vi "FGV Gasbottledefinition.vi"(6 "Aktion":T5, 8 "error in (no error)":errorcluster caption="Fehler (Eingang, kein Fehler)", 11 "Gasflasche Text Array":T3[](array[typedef])) -> (0 "error out":errorcluster caption="Fehler (Ausgang)", 2 "Gasflaschen Liste gesamt":T1[](array[typedef]) {"Gasflasche"."Ablaufdatum" format="%<%d.%m.%Y>T"; "Komponenten"."Konzentration IST" format="%#.4f"; "Komponenten"."Genauigkeit" format="%#.1f"}, 3 "Gasflaschen Text Liste gesamt":T3[][](array[typedef]))   [LabVIEW 2020, in "System Einstellungen V2.lvlib"]
uses:
  System Einstellungen V2.lvlib
  Aktion FGV Gasbottledefinition.ctl
  Traegergas.ctl
  Gasflasche gesamt.ctl
  Gasflasche.ctl
  Gasflaschenkomponente.ctl
  EPA 1065/Allgemeine VIs/Aktion Wertaenderung Gasliste.ctl
  Allgemein/allgemeine Sub-VIs.lvlib
  EPA 1065/EPA 1065.lvlib
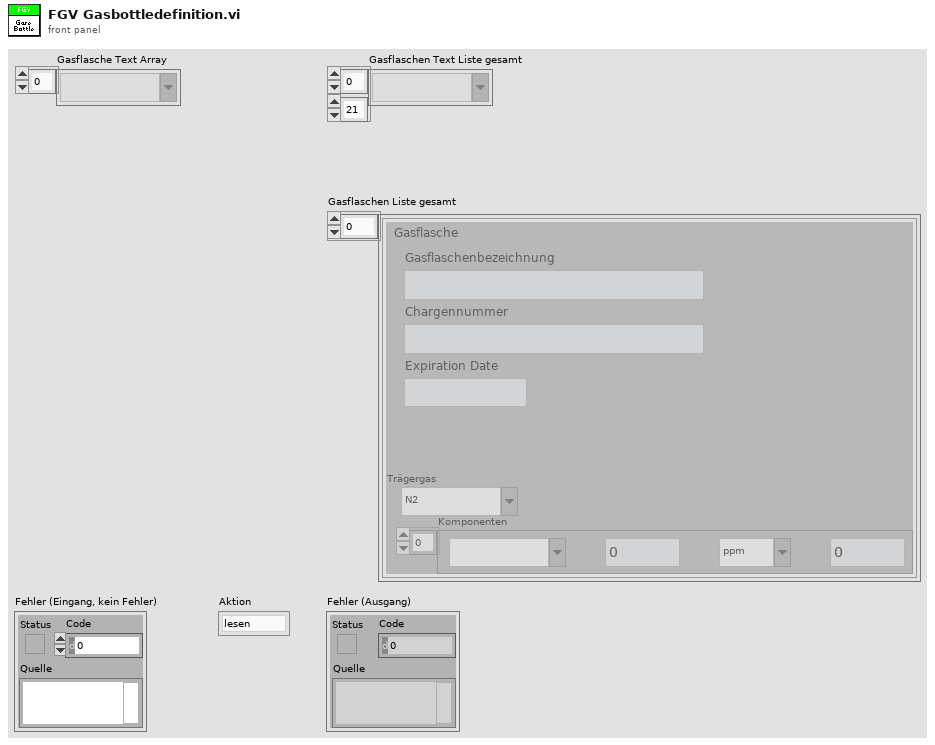
[diagram p1: front panel]
types:
  T1 = typedef "System Einstellungen V2.lvlib/Gasflasche gesamt.ctl" = cluster{"Gasflasche":T2, "Trägergas":T3, "Komponenten":T4[]}
  T2 = typedef "System Einstellungen V2.lvlib/Gasflasche.ctl" = cluster{"Gasname für die Auswahl":string, "Chargennummer":string, "Ablaufdatum":timestamp}
  T3 = typedef "System Einstellungen V2.lvlib/Traegergas.ctl" = string
  T4 = typedef "System Einstellungen V2.lvlib/Gasflaschenkomponente.ctl" = cluster{"Gasauswahl":string, "Konzentration IST":dbl, "Einheit":string, "Genauigkeit":dbl}
  T5 = typedef "System Einstellungen V2.lvlib/Aktion FGV Gasbottledefinition.ctl" = enum16{"lesen", "schreiben", "löschen", "laden", "speichern", "exportieren", "importieren"}
  T6 = typedef "EPA 1065.lvlib/Aktion Wertaenderung Gasliste.ctl" = enum16{"Init", "lesen", "Gasliste geändert", "ARN inaktiv", "LEAK inaktiv", "Interference 366 inaktiv", "T90 inaktiv", "Interference 375 inaktiv", "Chiller inaktiv", "FID O2 inaktiv", "FID Opti inaktiv", "Drift inaktiv", "Pre Test inaktiv", "LinV2 inaktiv"}
  T7 = enum16{"lesen", "schreiben", "löschen", "laden", "speichern"}
  T8 = enum16{"open", "replace", "create", "open or create", "replace or create", "replace or create with confirmation"}
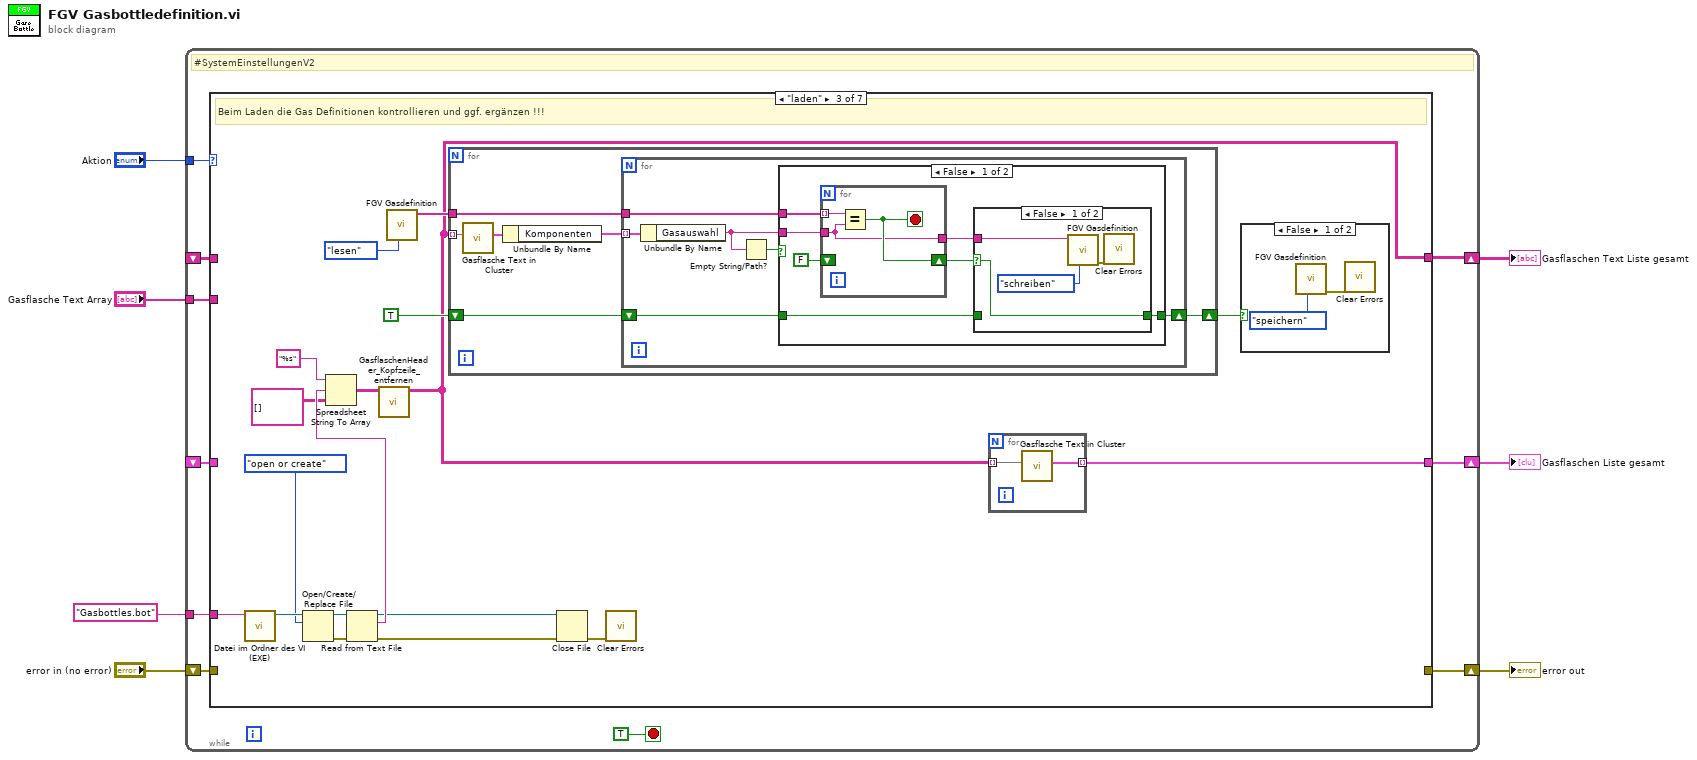
[diagram p0: block diagram]
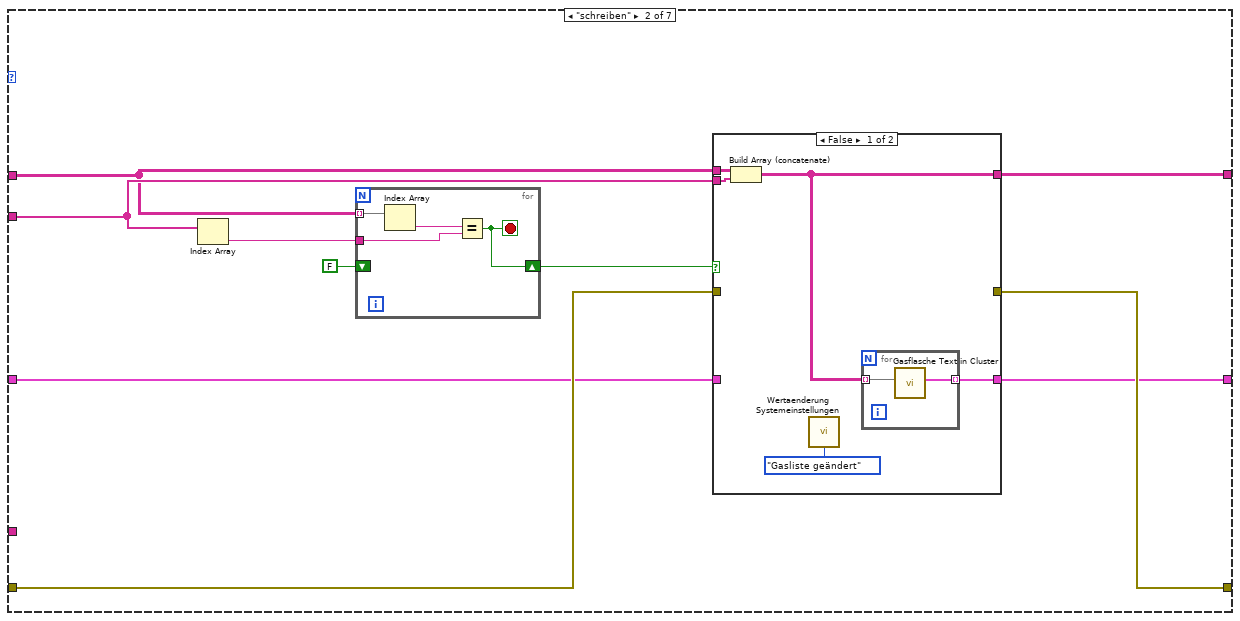
[diagram p3: hidden frame]
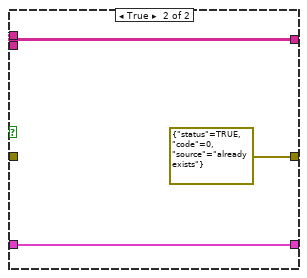
[diagram p4: hidden frame]
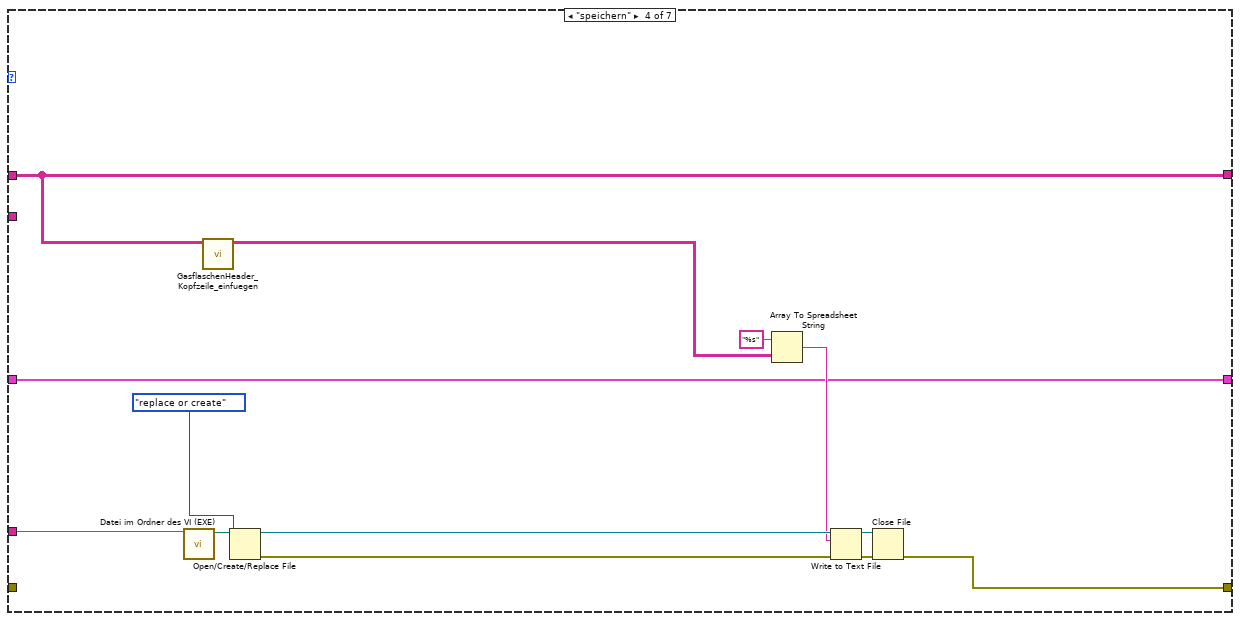
[diagram p8: hidden frame]
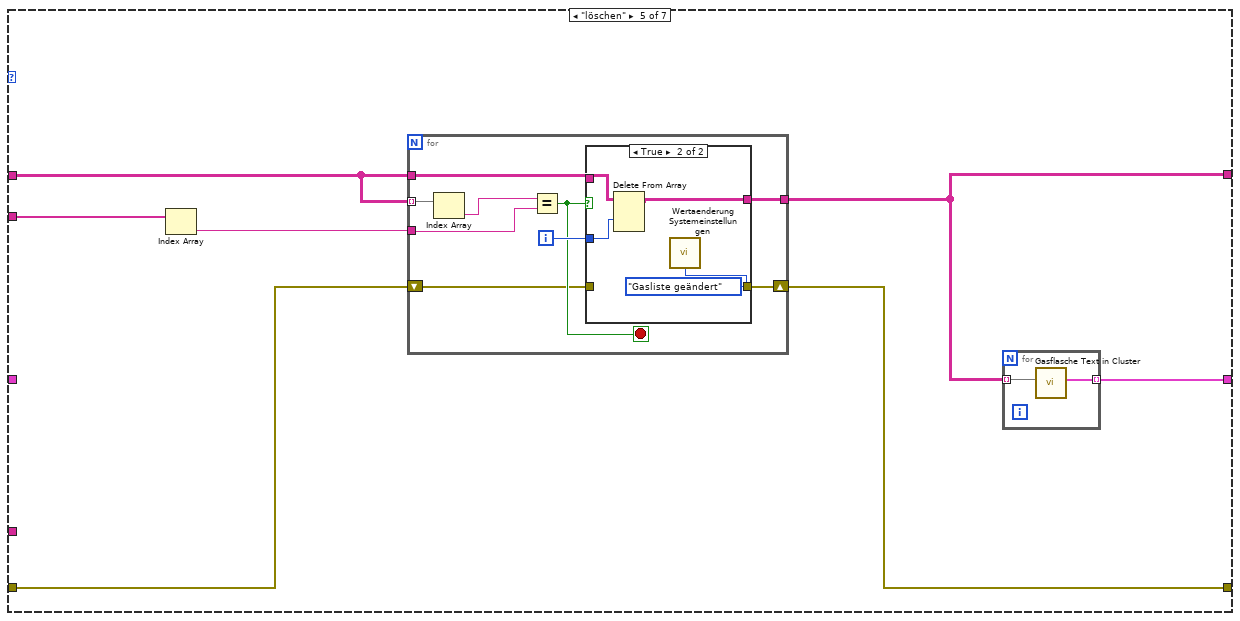
[diagram p9: hidden frame]
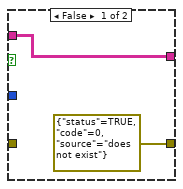
[diagram p10: hidden frame]
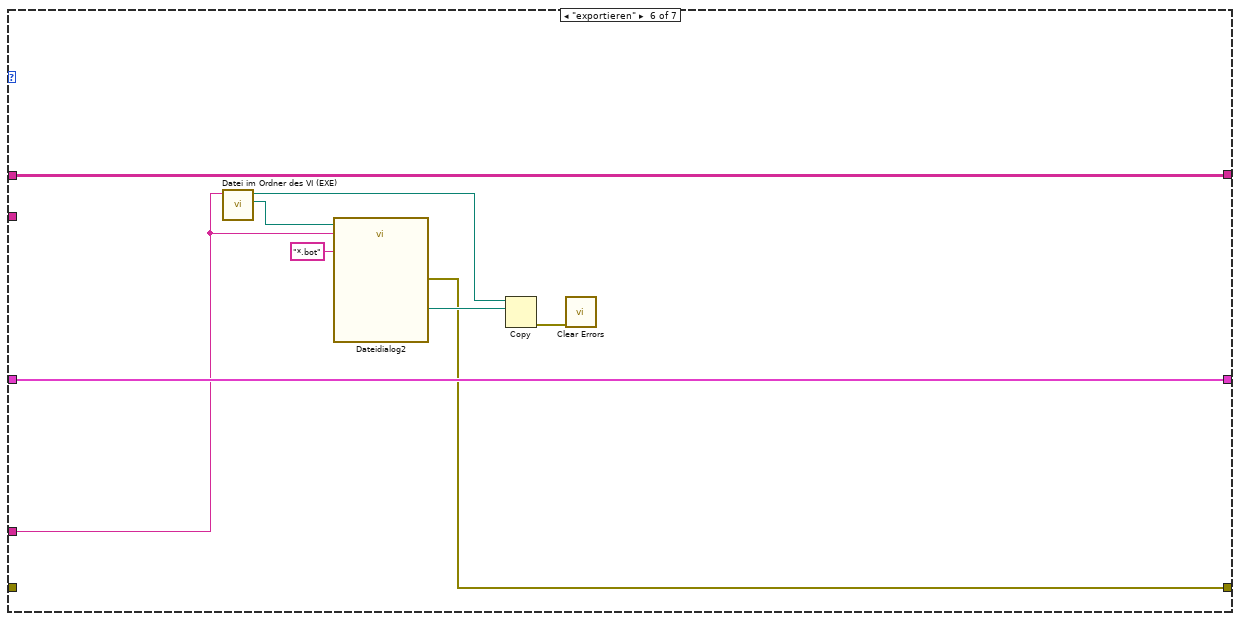
[diagram p11: hidden frame]
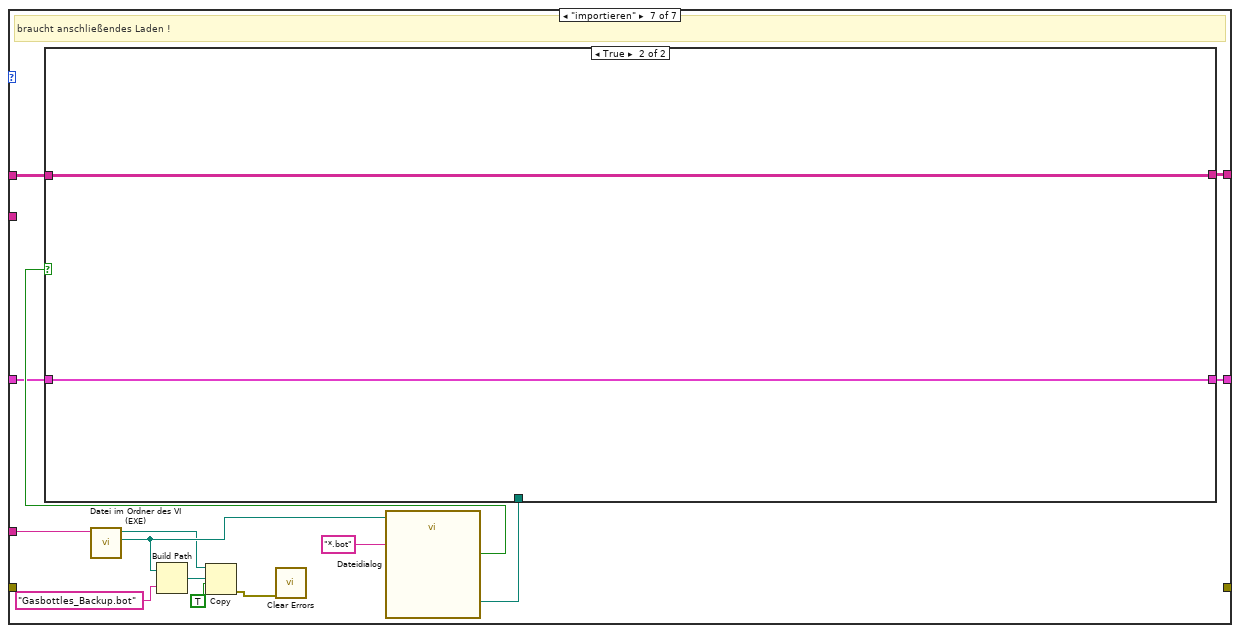
[diagram p12: hidden frame]
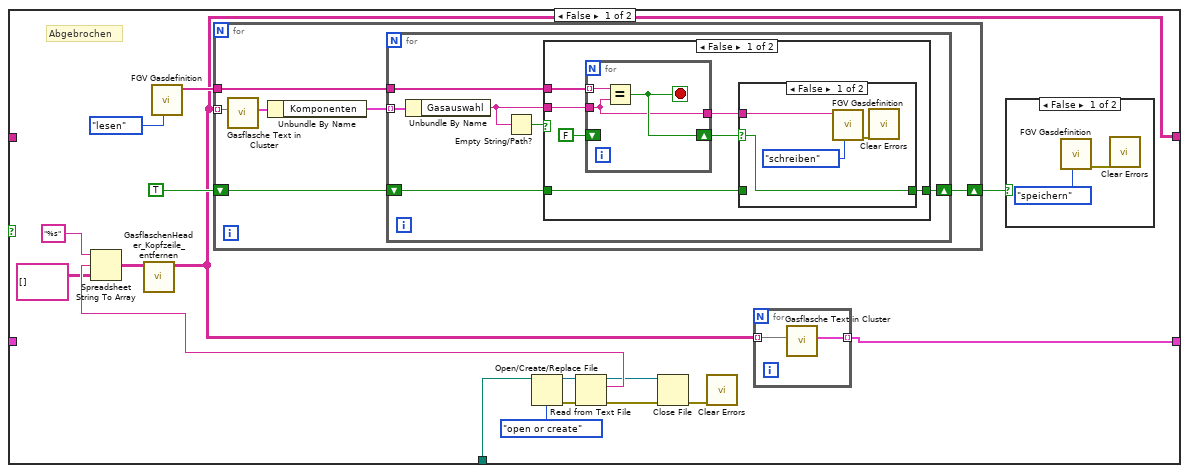
[diagram p13: hidden frame]
diagram:
  n1 = while {
    tunnel: "Aktion" -> [w16]
    shift-right: [w13] -> w2
    shift-left: _ -> [w15]
    tunnel: "Gasbottles.bot" ("Dateiname") -> [w14]
    tunnel: "Gasflasche Text Array" -> [w12]
    shift-right: [w10] -> w3
    shift-left: "error in (no error)" -> [w11]
    shift-right: [w9] -> w1
    shift-left: _ -> [w8]
    stop <- TRUE stop-if-true
    # "#SystemEinstellungenV2"
    n2 = case shown="\"laden\"" w16 {
      tunnel: [w19 w29 w45 w95 w108 w139 w151] -> w13
      tunnel: w15 -> [w19 w24 _ w95 w111 w139 w141]
      tunnel: w14 -> [_ _ w61 w105 _ w132 w153]
      tunnel: w12 -> [_ w26 _ _ w113 _ _]
      tunnel: w11 -> [_ w23 _ _ w110 _ _]
      tunnel: [_ w22 _ w97 w109 w133 _] -> w10
      tunnel: [w18 w21 w46 w96 w107 w138 w150] -> w9
      tunnel: w8 -> [w18 w20 _ w96 _ w138 w140]
      frame "lesen", Default {
      }
      frame "schreiben" {
        n3 = Index Array(array=w26) -> (element=w25:T3)  [unwired: 1 in]
        n4 = for {
          tunnel: w25 -> [w43]
          shift-right: [w42] -> w27
          shift-left: FALSE -> [_]
          tunnel: w24 -> [w41] mode=indexing
          stop <- w42 stop-if-true
          n5 = Index Array(array=w41) -> (element=w40:T3)  [unwired: 1 in]
          n6 = Equal?(x=w40, y=w43) -> (x = y?=w42:bool)
        }
        n7 = case shown="False" w27 {
          tunnel: [w32 w39] -> w29
          tunnel: w24 -> [w34 w39]
          tunnel: w26 -> [w33 _]
          tunnel: w23 -> [_ _]
          tunnel: [_ errorcluster {"status"=TRUE, "code"=0, "source"="already exists"} ("error in (no error)")] -> w22
          tunnel: [w31 w37] -> w21
          tunnel: w20 -> [_ w37]
          frame False {
            n8 = Build Array (concatenate)(w34, w33) -> (w32:T3[][])
            n9 = call "Wertaenderung Systemeinstellungen.vi"("Aktion"=Aktion_Wertaenderung_Gasliste."Gasliste geändert") -> ()  [unwired: 13 in, 2 out]
            n10 = for {
              tunnel: w32 -> [w36] mode=indexing
              tunnel: [w35] -> w31 mode=indexing
              n11 = call "Gasflasche Text in Cluster.vi"("Gasflasche Text Array"=w36) -> ("Gasflasche"=w35:T1)  [unwired: 10 in]
            }
          }
          frame True {
          }
        }
      }
      frame "laden" {
        # "Beim Laden die Gas Definitionen kontrollieren und ggf. ergänzen !!!"
        n12 = call "Datei im Ordner des VI (EXE).vi"("Dateiname"=w61) -> ("Dateipfad im Ordner des Haupt-VIs"=w60:path)  [unwired: 8 in, 2 out]
        n13 = Open/Create/Replace File(file path (use dialog)=w60, operation (0:open)=T8."open or create" ("Operation (0:open)")) -> (refnum out=w58:refnum<file>, error out=w59:errorcluster)  [unwired: 4 in, 1 out]
        n14 = Read from Text File(file (use dialog)=w58, error in=w59) -> (refnum out=w54:refnum<file>, text=w57:string, error out=w53:errorcluster)  [unwired: 2 in, 1 out]
        n15 = Spreadsheet String To Array(format string="%s" ("Format-String"), spreadsheet string=w57, array type (2D Dbl)=string[][] []) -> (array=w44:string[][])  [unwired: 1 in]
        n16 = call "GasflaschenHeader_Kopfzeile_entfernen.vi"("Array (Eingang)"=w44) -> ("Array (Ausgang)"=w45:string[][])  [unwired: 10 in]
        n17 = call "FGV Gasdefinition.vi"("Aktion"=T7."lesen") -> ("Gase"=w49:string[])  [unwired: 9 in, 1 out]
        n18 = for {
          tunnel: w45 -> [w68] mode=indexing
          tunnel: w49 -> [w71]
          shift-right: [w69] -> w47
          shift-left: TRUE -> [w70]
          n19 = call "Gasflasche Text in Cluster.vi"("Gasflasche Text Array"=w68) -> ("Gasflasche"=w67:T1)  [unwired: 10 in]
          n20 = Unbundle By Name(w67) -> ("Komponenten"=w66:T4[])
          n21 = for {
            tunnel: w71 -> [w77]
            tunnel: w66 -> [w74] mode=indexing
            shift-right: [w75] -> w69
            shift-left: w70 -> [w76]
            n22 = Unbundle By Name(w74) -> ("Gasauswahl"=w72:string)
            n23 = Empty String/Path?(string/path=w72) -> (empty?=w73:bool)
            n24 = case shown="False" w73 {
              tunnel: w77 -> [w84 _]
              tunnel: w76 -> [w80 w93]
              tunnel: [w79 w93] -> w75
              tunnel: w72 -> [w78 _]
              frame False {
                n25 = for {
                  tunnel: w84 -> [w92] mode=indexing
                  tunnel: w78 -> [w90]
                  shift-right: [w91] -> w81
                  shift-left: FALSE -> [_]
                  tunnel: [w90] -> w82
                  stop <- w91 stop-if-true
                  n26 = Equal?(x=w92, y=w90) -> (x = y?=w91:bool)
                }
                n27 = case shown="False" w81 {
                  selector: w81 -> [w86 _]
                  tunnel: w82 -> [w87 _]
                  tunnel: w80 -> [_ w89]
                  tunnel: [w86 w89] -> w79
                  frame False {
                    n28 = call "FGV Gasdefinition.vi"("Aktion"=T7."schreiben", "Gas"=w87) -> ("error out"=w85:errorcluster)  [unwired: 8 in, 1 out]
                    n29 = call <vilib>:"Clear Errors.vi"("error in (no error)"=w85) -> ()  [unwired: 5 in, 2 out]
                  }
                  frame True {
                  }
                }
              }
              frame True {
              }
            }
          }
        }
        n30 = Close File(refnum=w54, error in=w53) -> (error out=w55:errorcluster)  [unwired: 1 out]
        n31 = call <vilib>:"Clear Errors.vi"("error in (no error)"=w55) -> ()  [unwired: 5 in, 2 out]
        n32 = for {
          tunnel: w45 -> [w63] mode=indexing
          tunnel: [w62] -> w46 mode=indexing
          n33 = call "Gasflasche Text in Cluster.vi"("Gasflasche Text Array"=w63) -> ("Gasflasche"=w62:T1)  [unwired: 10 in]
        }
        n34 = case shown="False" w47 {
          frame False {
            n35 = call "FGV Gasdefinition.vi"("Aktion"=T7."speichern") -> ("error out"=w64:errorcluster)  [unwired: 9 in, 1 out]
            n36 = call <vilib>:"Clear Errors.vi"("error in (no error)"=w64) -> ()  [unwired: 5 in, 2 out]
          }
          frame True {
          }
        }
      }
      frame "speichern" {
        n37 = call "Datei im Ordner des VI (EXE).vi"("Dateiname"=w105) -> ("Dateipfad im Ordner des Haupt-VIs"=w106:path)  [unwired: 8 in, 2 out]
        n38 = call "GasflaschenHeader_Kopfzeile_einfuegen.vi"("Array (Eingang)"=w95) -> ("Array (Ausgang)"=w94:T3[][])  [unwired: 10 in]
        n39 = Open/Create/Replace File(file path (use dialog)=w106, operation (0:open)=T8."replace or create" ("Operation (0:open)")) -> (refnum out=w104:refnum<file>, error out=w103:errorcluster)  [unwired: 4 in, 1 out]
        n40 = Array To Spreadsheet String(array=w94, 3:"%s" ("Format-String")) -> (spreadsheet string=w100:string)  [unwired: 1 in]
        n41 = Write to Text File(file (use dialog)=w104, text=w100, error in=w103) -> (refnum out=w101:refnum<file>, error out=w102:errorcluster)  [unwired: 1 in, 1 out]
        n42 = Close File(refnum=w101, error in=w102) -> (error out=w97:errorcluster)  [unwired: 1 out]
      }
      frame "löschen" {
        n43 = Index Array(array=w113) -> (element=w112:T3)  [unwired: 1 in]
        n44 = for {
          tunnel: w112 -> [w124]
          tunnel: w111 -> [w123]
          tunnel: [w121] -> w108
          tunnel: w111 -> [w119] mode=indexing
          shift-right: [w116] -> w109
          shift-left: w110 -> [w117]
          i -> [w122]
          stop <- w120 stop-if-true
          n45 = Index Array(array=w119) -> (element=w118:T3)  [unwired: 1 in]
          n46 = Equal?(x=w118, y=w124) -> (x = y?=w120:bool)
          n47 = case shown="True" w120 {
            tunnel: w123 -> [w126 w130]
            tunnel: w122 -> [_ w129]
            tunnel: [w126 w128] -> w121
            tunnel: w117 -> [_ _]
            tunnel: [errorcluster {"status"=TRUE, "code"=0, "source"="does not exist"} ("error in (no error)") _] -> w116
            frame False {
            }
            frame True {
              n48 = Delete From Array(array=w130, index (row)=w129) -> (array with subset deleted=w128:T3[][])  [unwired: 2 in, 1 out]
              n49 = call "Wertaenderung Systemeinstellungen.vi"("Aktion"=Aktion_Wertaenderung_Gasliste."Gasliste geändert") -> ()  [unwired: 13 in, 2 out]
            }
          }
        }
        n50 = for {
          tunnel: w108 -> [w115] mode=indexing
          tunnel: [w114] -> w107 mode=indexing
          n51 = call "Gasflasche Text in Cluster.vi"("Gasflasche Text Array"=w115) -> ("Gasflasche"=w114:T1)  [unwired: 10 in]
        }
      }
      frame "exportieren" {
        n52 = call "Datei im Ordner des VI (EXE).vi"("Dateiname"=w132) -> ("Ordner des Haupt-VIs"=w137:path, "Dateipfad im Ordner des Haupt-VIs"=w135:path)  [unwired: 8 in, 1 out]
        n53 = call "Dateidialog2"("start path"=w137, "default name"=w132, "pattern (all files)"="*.bot") -> ("selected path"=w134:path, "error out"=w133:errorcluster)  [unwired: 9 in, 2 out]
        n54 = Copy(10:w134, 11:w135) -> (0:w131:errorcluster)  [unwired: 3 in, 2 out]
        n55 = call <vilib>:"Clear Errors.vi"("error in (no error)"=w131) -> ()  [unwired: 5 in, 2 out]
      }
      frame "importieren" {
        # "braucht anschließendes Laden !"
        n56 = call "Datei im Ordner des VI (EXE).vi"("Dateiname"=w153) -> ("Ordner des Haupt-VIs"=w148:path, "Dateipfad im Ordner des Haupt-VIs"=w143:path)  [unwired: 8 in, 1 out]
        n57 = Build Path(base path=w148, name or relative path="Gasbottles_Backup.bot" ("Dateiname")) -> (appended path=w146:path)
        n58 = Copy(9:TRUE ("Überschreiben (F)"), 10:w146, 11:w143) -> (0:w144:errorcluster)  [unwired: 2 in, 2 out]
        n59 = call <vilib>:"Clear Errors.vi"("error in (no error)"=w144) -> ()  [unwired: 5 in, 2 out]
        n60 = call "Dateidialog"("start path"=w148, "pattern (all files)"="*.bot") -> ("selected path"=w149:path, "cancelled"=w142:bool)  [unwired: 10 in, 2 out]
        n61 = case shown="True" w142 {
          tunnel: [w156 w204] -> w151
          tunnel: [w155 w203] -> w150
          tunnel: w149 -> [w154 _]
          tunnel: w141 -> [_ w204]
          tunnel: w140 -> [_ w203]
          frame False {
            # "Abgebrochen"
            n62 = call "FGV Gasdefinition.vi"("Aktion"=T7."lesen") -> ("Gase"=w160:string[])  [unwired: 9 in, 1 out]
            n63 = Open/Create/Replace File(file path (use dialog)=w154, operation (0:open)=T8."open or create" ("Operation (0:open)")) -> (refnum out=w169:refnum<file>, error out=w170:errorcluster)  [unwired: 4 in, 1 out]
            n64 = Read from Text File(file (use dialog)=w169, error in=w170) -> (refnum out=w165:refnum<file>, text=w168:string, error out=w164:errorcluster)  [unwired: 2 in, 1 out]
            n65 = Spreadsheet String To Array(format string="%s" ("Format-String"), spreadsheet string=w168, array type (2D Dbl)=string[][] []) -> (array=w157:string[][])  [unwired: 1 in]
            n66 = call "GasflaschenHeader_Kopfzeile_entfernen.vi"("Array (Eingang)"=w157) -> ("Array (Ausgang)"=w156:string[][])  [unwired: 10 in]
            n67 = for {
              tunnel: w156 -> [w177] mode=indexing
              tunnel: w160 -> [w180]
              shift-right: [w178] -> w158
              shift-left: TRUE -> [w179]
              n68 = call "Gasflasche Text in Cluster.vi"("Gasflasche Text Array"=w177) -> ("Gasflasche"=w176:T1)  [unwired: 10 in]
              n69 = Unbundle By Name(w176) -> ("Komponenten"=w175:T4[])
              n70 = for {
                tunnel: w180 -> [w186]
                tunnel: w175 -> [w183] mode=indexing
                shift-right: [w184] -> w178
                shift-left: w179 -> [w185]
                n71 = Unbundle By Name(w183) -> ("Gasauswahl"=w181:string)
                n72 = Empty String/Path?(string/path=w181) -> (empty?=w182:bool)
                n73 = case shown="False" w182 {
                  tunnel: w186 -> [w193 _]
                  tunnel: w185 -> [w189 w202]
                  tunnel: [w188 w202] -> w184
                  tunnel: w181 -> [w187 _]
                  frame False {
                    n74 = for {
                      tunnel: w193 -> [w201] mode=indexing
                      tunnel: w187 -> [w199]
                      shift-right: [w200] -> w190
                      shift-left: FALSE -> [_]
                      tunnel: [w199] -> w191
                      stop <- w200 stop-if-true
                      n75 = Equal?(x=w201, y=w199) -> (x = y?=w200:bool)
                    }
                    n76 = case shown="False" w190 {
                      selector: w190 -> [w195 _]
                      tunnel: w191 -> [w196 _]
                      tunnel: w189 -> [_ w198]
                      tunnel: [w195 w198] -> w188
                      frame False {
                        n77 = call "FGV Gasdefinition.vi"("Aktion"=T7."schreiben", "Gas"=w196) -> ("error out"=w194:errorcluster)  [unwired: 8 in, 1 out]
                        n78 = call <vilib>:"Clear Errors.vi"("error in (no error)"=w194) -> ()  [unwired: 5 in, 2 out]
                      }
                      frame True {
                      }
                    }
                  }
                  frame True {
                  }
                }
              }
            }
            n79 = Close File(refnum=w165, error in=w164) -> (error out=w166:errorcluster)  [unwired: 1 out]
            n80 = call <vilib>:"Clear Errors.vi"("error in (no error)"=w166) -> ()  [unwired: 5 in, 2 out]
            n81 = for {
              tunnel: w156 -> [w172] mode=indexing
              tunnel: [w171] -> w155 mode=indexing
              n82 = call "Gasflasche Text in Cluster.vi"("Gasflasche Text Array"=w172) -> ("Gasflasche"=w171:T1)  [unwired: 10 in]
            }
            n83 = case shown="False" w158 {
              frame False {
                n84 = call "FGV Gasdefinition.vi"("Aktion"=T7."speichern") -> ("error out"=w173:errorcluster)  [unwired: 9 in, 1 out]
                n85 = call <vilib>:"Clear Errors.vi"("error in (no error)"=w173) -> ()  [unwired: 5 in, 2 out]
              }
              frame True {
              }
            }
          }
          frame True {
          }
        }
      }
    }
  }
  "error out" <- w3
  "Gasflaschen Text Liste gesamt" <- w2
  "Gasflaschen Liste gesamt" <- w1
